vi "LogRobotPositionData.vi"(8 "Iterations between saves":i32=10, 9 "Iteration counter":i32, 10 "Global Robot Data":T1, 11 "Datalog File Refnum in":refnum<k34>) -> (3 "Datalog File Refnum out":refnum<k34>)   [LabVIEW 2014]
uses:
  Variables/Default global.vi
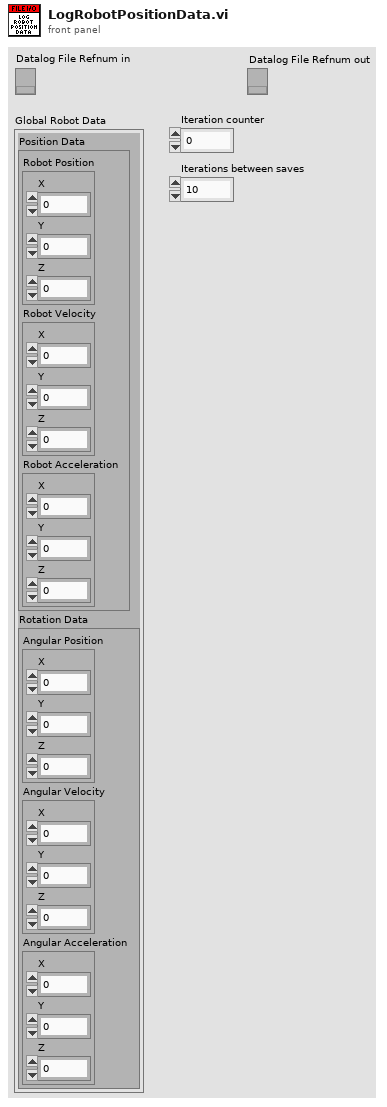
[diagram p1: front panel]
types:
  T1 = cluster{"Position Data":cluster{"Robot Position":cluster{"X":dbl, "Y":dbl, "Z":dbl}, "Robot Velocity":cluster{"X":dbl, "Y":dbl, "Z":dbl}, "Robot Acceleration":cluster{"X":dbl, "Y":dbl, "Z":dbl}}, "Rotation Data":cluster{"Angular Position":cluster{"X":dbl, "Y":dbl, "Z":dbl}, "Angular Velocity":cluster{"X":dbl, "Y":dbl, "Z":dbl}, "Angular Acceleration":cluster{"X":dbl, "Y":dbl, "Z":dbl}}}
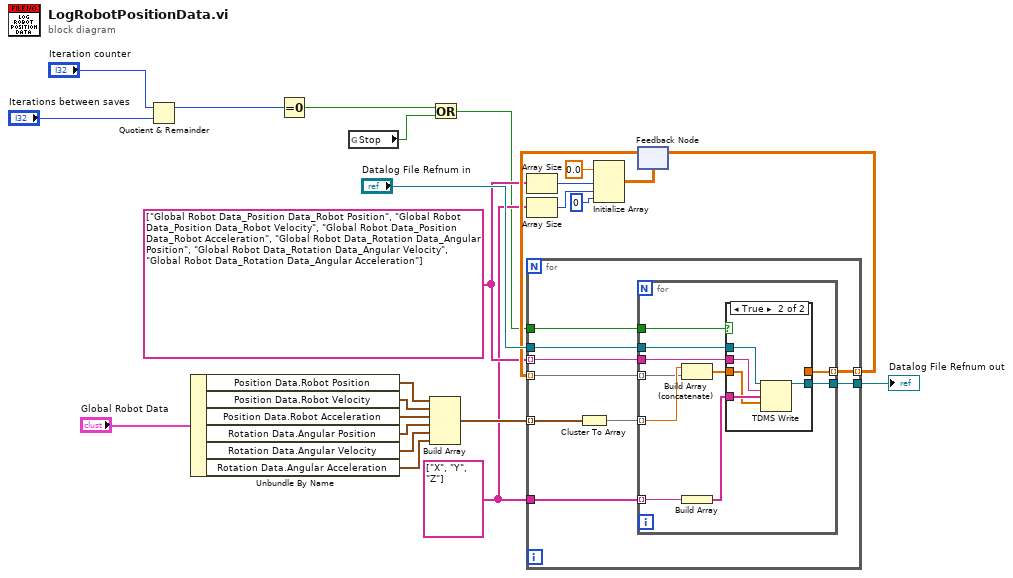
[diagram p0: block diagram]
diagram:
  w10 = string[] ["X", "Y", "Z"] ("Array of Channels")
  w11 = string[] ["Global Robot Data_Position Data_Robot Position", "Global Robot Data_Position Data_Robot Velocity", "Global Robot Data_Position Data_Robot Acceleration", "Global Robot Data_Rotation Data_Angular Position", "Global Robot Data_Rotation Data_Angular Velocity", "Global Robot Data_Rotation Data_Angular Acceleration"] ("Array of Channels")
  n1 = Quotient & Remainder(x="Iteration counter", y="Iterations between saves") -> (x-y*floor(x/y)=w4:i32)  [unwired: 1 out]
  n2 = Unbundle By Name("Global Robot Data") -> ("Position Data.Robot Position"=w18:cluster{"X":dbl, "Y":dbl, "Z":dbl}, "Position Data.Robot Velocity"=w19:cluster{"X":dbl, "Y":dbl, "Z":dbl}, "Position Data.Robot Acceleration"=w20:cluster{"X":dbl, "Y":dbl, "Z":dbl}, "Rotation Data.Angular Position"=w21:cluster{"X":dbl, "Y":dbl, "Z":dbl}, "Rotation Data.Angular Velocity"=w22:cluster{"X":dbl, "Y":dbl, "Z":dbl}, "Rotation Data.Angular Acceleration"=w23:cluster{"X":dbl, "Y":dbl, "Z":dbl})
  n3 = Equal To 0?(x=w4) -> (x = 0?=w3:bool)
  n4 = global read "Default global.vi" "Stop"() -> (w2:bool)
  n5 = Build Array(w18, w19, w20, w21, w22, w23) -> (w24:cluster{"X":dbl, "Y":dbl, "Z":dbl}[])
  n6 = Or(x=w3, y=w2) -> (x .or. y?=w1:bool)
  n7 = Array Size(array=w11) -> (size(s)=w9:i32)
  n8 = Array Size(array=w10) -> (size(s)=w8:i32)
  n9 = Initialize Array(0.0 ("element"), w9, w8, 0 ("dimension size")) -> (w12:dbl[][][])
  n10 = feedback #1(w12) -> (w14:dbl[][][])
  n11 = for {
    tunnel: w24 -> [w34] mode=indexing
    tunnel: w11 -> [w33] mode=indexing
    tunnel: "Datalog File Refnum in" -> [w32]
    tunnel: [w30] -> w17
    tunnel: [w29] -> w15 mode=indexing
    tunnel: w14 -> [w28] mode=indexing
    tunnel: w10 -> [w27]
    tunnel: w1 -> [w26]
    n12 = Cluster To Array(cluster=w34) -> (array=w31:dbl[])
    n13 = for {
      tunnel: w31 -> [w39] mode=indexing
      tunnel: w27 -> [w41] mode=indexing
      tunnel: w33 -> [w44]
      tunnel: w32 -> [w43]
      tunnel: [w42] -> w30
      tunnel: [w37] -> w29 mode=indexing
      tunnel: w28 -> [w36] mode=indexing
      tunnel: w26 -> [w35]
      n14 = Build Array (concatenate)(w39, w36) -> (w38:dbl[])
      n15 = Build Array(w41) -> (w40:string[])
      n16 = case shown="True" w35 {
        tunnel: w44 -> [_ w51]
        tunnel: w43 -> [w46 w50]
        tunnel: [w46 w49] -> w42
        tunnel: w40 -> [_ w48]
        tunnel: w38 -> [w45 w47]
        tunnel: [w45 _] -> w37
        frame False {
        }
        frame True {
          n17 = TDMS Write(0:w50, 5:w51, 7:w48, 9:w47) -> (4:w49:refnum<k34>)  [unwired: 2 in, 3 out]
        }
      }
    }
  }
  "Datalog File Refnum out" <- w17
  n18 = feedback-in #1(w15) -> ()
